vi "findNewLocation_Jiggle.vi"(6 "mazeDirection":string, 8 "error in (no error)":errorcluster, 9 "up or down":string, 10 "possible \nlocations":dbl[](array[numeric]), 11 "start \nlocation":dbl[](array[numeric])) -> (0 "error out":errorcluster, 3 "new\nplatform":i32)   [LabVIEW 2017]
uses:
  <vilib>/Utility/error.llb/DialogType.ctl
panel:
  out "Animals location":string
  out "message":string=" INSTRUCTIONS:\r\rNormal Use:  When using subVIs that incorporate the error in/error out (or error I/O) structure, place this handler where you want to inform the user of an error, typically at the end of the I/O data path, as the last action of the program.  If the error in error? is ERROR, the handler creates a message describing the error and its source.  If the type of dialog = 1 (default), the message is displayed to the user, who can only acknowedge it.  If the type = 2, the user can acknowledge the message or abort execution; aborting a program with active I/O is not recommended.  If the type = 0, no message is displayed; this is used to process the error programmatically, and the error out cluster elements are wired to individual terminals for that reason.  \r\rOther Use:\n\r\nlocal testing.  To test the error code of a subVI or function that does not have the error I/O structure, you can wire its error code and a source string to the local error code and error source inputs.  If error in error? indicates no error and error code is not equal to 0, the local code and source are substituted for the error in values, and error? is set TRUE (ERROR)."
  out "source out":string
  out "code out":i32 format="%0.0f"
  out "error?":bool
  in  "type of dialog (OK msg:1)":T1=1 items=["no dialog", "OK message", "continue or stop message", "OK message + warnings", "continue/stop + warnings"]
  in  "error source (\" \")":string
  in  "error code (no error:0)":i32 format="%0.0f"
  in  "delay":dbl=4000.0
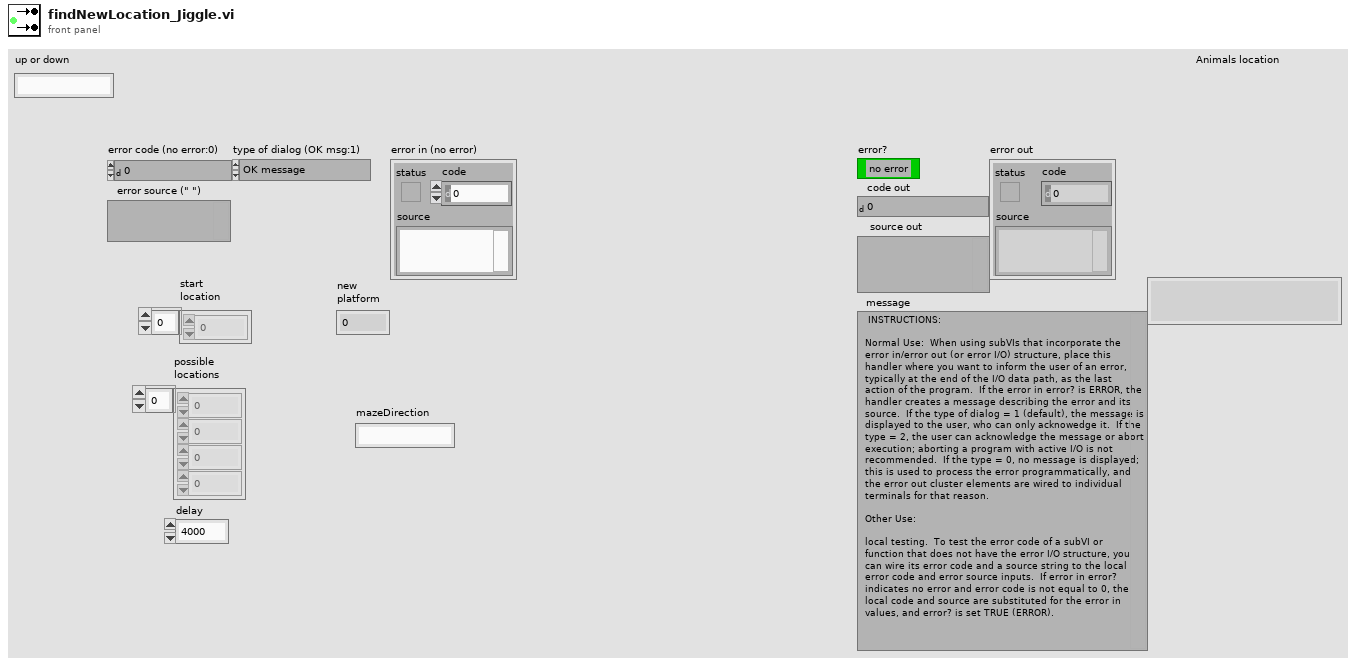
[diagram p1: front panel]
types:
  T1 = typedef "DialogType.ctl" = u16
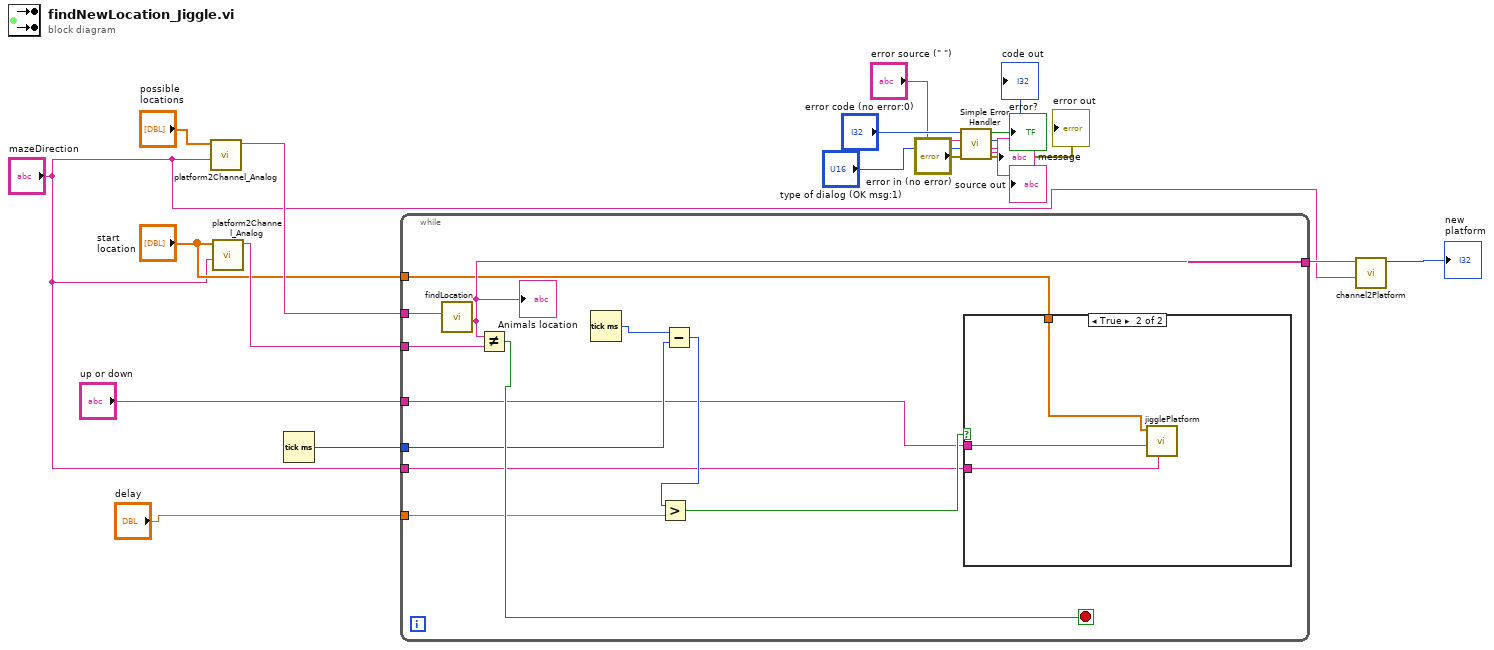
[diagram p0: block diagram]
diagram:
  n1 = call "platform2Channel_Analog.vi"("mazeDirection"="mazeDirection", "platforms"="possible \nlocations") -> ("DAQmx Channel"=w17:string)  [unwired: 9 in]
  n2 = call "platform2Channel_Analog.vi"("mazeDirection"="mazeDirection", "platforms"="start \nlocation") -> ("DAQmx Channel"=w16:string)  [unwired: 9 in]
  n3 = Tick Count (ms)() -> (millisecond timer value=w14:u32)
  n4 = while {
    tunnel: w17 -> [w31]
    tunnel: w16 -> [w30]
    tunnel: [w29] -> w15
    tunnel: w14 -> [w26]
    tunnel: "start \nlocation" -> [w24]
    tunnel: "delay" -> [w22]
    tunnel: "up or down" -> [w21]
    tunnel: "mazeDirection" -> [w20]
    stop <- w28 stop-if-true
    n5 = call "findLocation.vi"("DAQmx \nPhysical Channel"=w31) -> ("Animals location"=w29:string)  [unwired: 10 in]
    "Animals location" <- w29
    n6 = Not Equal?(x=w29, y=w30) -> (x != y?=w28:bool)
    n7 = Tick Count (ms)() -> (millisecond timer value=w27:u32)
    n8 = Subtract(x=w27, y=w26) -> (x-y=w25:u32)
    n9 = Greater?(x=w25, y=w22) -> (0:w23:bool)
    n10 = case shown="True" w23 {
      tunnel: w24 -> [_ w34]
      tunnel: w21 -> [_ w33]
      tunnel: w20 -> [_ w32]
      frame False {
      }
      frame True {
        n11 = call "jigglePlatform.vi"("mazeDirection"=w32, "up or down"=w33, "Platforms\nto jiggle"=w34) -> ()  [unwired: 9 in]
      }
    }
  }
  n12 = call <vilib>:"Simple Error Handler.vi"("error code (no error:0)"="error code (no error:0)", "error source (\" \")"="error source (\" \")", "type of dialog (OK msg:1)"="type of dialog (OK msg:1)", "error in (no error)"="error in (no error)") -> ("error?"=→"error?":bool, "code out"=→"code out":i32, "source out"=→"source out":string, "error out"=→"error out":errorcluster, "message"=→"message":string)  [unwired: 1 in]
  n13 = call "channel2Platform.vi"("mazeDirection"="mazeDirection", "DAQmx \nPhysical Channel"=w15) -> ("Platform number"=→"new\nplatform":i32)  [unwired: 9 in]
